vi "RSZVB Get Analyzer Hostname.vi"(8 "error in (no error)":errorcluster {"code" format="%.0x"}, 11 "VISA session":refnum<visa-resource-name>) -> (0 "error out":errorcluster {"code" format="%.0x"}, 2 "Host Name":string, 3 "dup VISA session":refnum<visa-resource-name>)   [LabVIEW 2011]
doc: "This VI queries the analyzer's host name (computer name). The domain is not included. \n\nRemote-control command(s):\nSYSTem:COMMunicate:NET:HOSTname?"
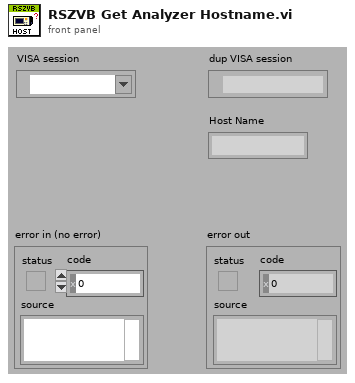
[diagram p1: front panel]
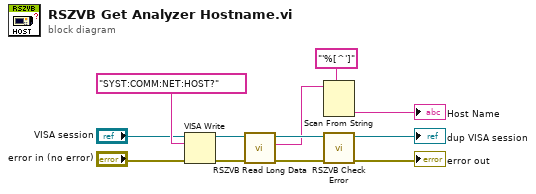
[diagram p0: block diagram]
diagram:
  n1 = VISA Write(VISA resource name="VISA session", write buffer="SYST:COMM:NET:HOST?", error in (no error)="error in (no error)") -> (VISA resource name out=w10:refnum<visa-resource-name>, error out=w9:errorcluster)  [unwired: 1 out]
  n2 = call "RSZVB Read Long Data.vi"("error in (no error)"=w9, "VISA resource name"=w10) -> ("error out"=w6:errorcluster, "Data"=w7:string, "VISA resource name out"=w8:refnum<visa-resource-name>)  [unwired: 7 in]
  n3 = Scan From String(format string="'%[^']", input string=w7) -> (output 1=→"Host Name":string)  [unwired: 3 in, 3 out]
  n4 = call "RSZVB Check Error.vi"("error in (no error)"=w6, "VISA session"=w8) -> ("error out"=→"error out":errorcluster, "dup VISA session"=→"dup VISA session":refnum<visa-resource-name>)  [unwired: 8 in]
